vi "AutoWfmToSpreadsheet_2019.vi"() -> ()   [LabVIEW 2019]
uses:
  <vilib>/Waveform/WDTFileIO.llb/Read Waveform from File.vi
  <vilib>/Waveform/WDTOps.llb/WDT Index Channel DBL.vi
  <vilib>/Waveform/WDTFileIO.llb/Export Waveforms To Spreadsheet File (1D).vi
panel:
  out "?":string
  in  "Path":i32
  in  "Path":string[](array[string])
  out "?":string
  out "Sinal adquirido":waveform(dbl)(graph)
  in  "?":bool
  in  "Escolher arquivo":i32
  out "Sinal de Referência":waveform(dbl)(graph)
  in  "V para Exportar/ F para Visualizar":bool
  out "result string":string
  out "element":string
  out "Numeric":i32
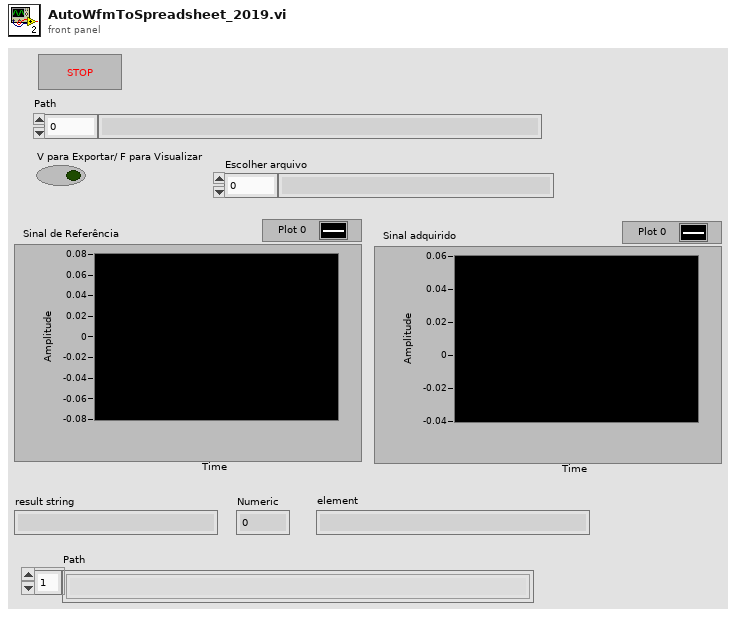
[diagram p1: front panel]
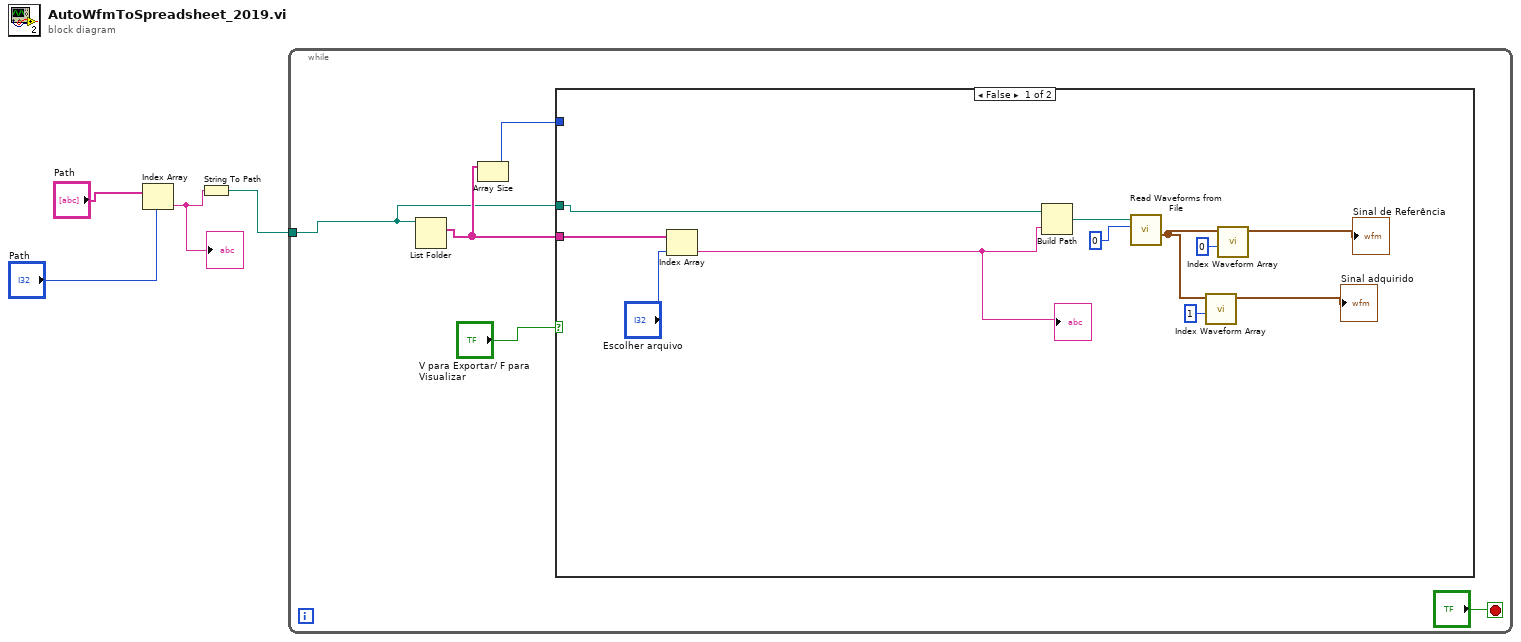
[diagram p0: block diagram]
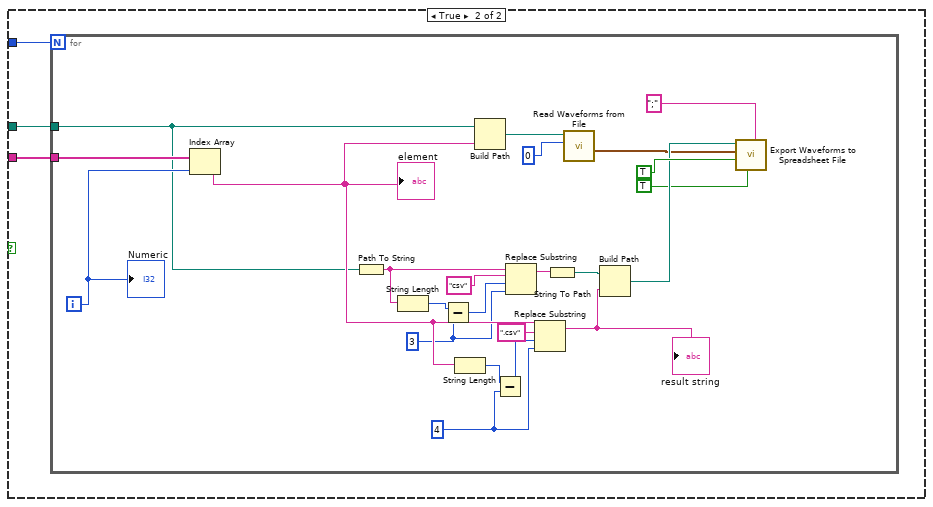
[diagram p2: hidden frame]
diagram:
  n1 = Index Array(array="Path", index="Path") -> (element=w1:string)
  "?" <- w1
  n2 = String To Path(string=w1) -> (path=w4:path)
  n3 = while {
    tunnel: w4 -> [w5]
    stop <- "?" stop-if-true
    n4 = List Folder(path=w5) -> (filenames=w9:string[])  [unwired: 3 in, 3 out]
    n5 = Array Size(array=w9) -> (size(s)=w8:i32)
    n6 = case shown="False" "V para Exportar/ F para Visualizar" {
      tunnel: w9 -> [w18 w23]
      tunnel: w8 -> [_ w22]
      tunnel: w5 -> [w10 w21]
      frame False {
        n7 = Index Array(array=w18, index="Escolher arquivo") -> (element=w13:string)
        "?" <- w13
        n8 = Build Path(base path=w10, name or relative path=w13) -> (appended path=w20:path)
        n9 = call-poly <vilib>:"Read Waveforms from File.vi"("offset (records:0)"=0, "file path (dialog if empty)"=w20) -> ("all waveforms in record"=w14:waveform(dbl)[])  [unwired: 4 in, 3 out]
        n10 = call-poly <vilib>:"Index Waveform Array.vi"("index"=1, "waveform array"=w14) -> ("waveform"=→"Sinal adquirido":waveform(dbl))  [unwired: 8 in, 1 out]
        n11 = call-poly <vilib>:"Index Waveform Array.vi"("index"=0, "waveform array"=w14) -> ("waveform"=→"Sinal de Referência":waveform(dbl))  [unwired: 8 in, 1 out]
      }
      frame True {
        n12 = for {
          N: w22 -> [_]
          tunnel: w23 -> [w46]
          tunnel: w21 -> [w31]
          i -> [w45]
          w26 = 3 ("y")
          w35 = 4 ("length (len. of substring)")
          n13 = Index Array(array=w46, index=w45) -> (element=w36:string)
          "element" <- w36
          n14 = Path To String(path=w31) -> (string=w29:string)
          n15 = String Length(string=w29) -> (length=w28:i32)
          n16 = Subtract(x=w28, y=w26) -> (x-y=w27:i32)
          n17 = String Length(string=w36) -> (length=w34:i32)
          n18 = Build Path(base path=w31, name or relative path=w36) -> (appended path=w43:path)
          n19 = Subtract(x=w34, y=w35) -> (x-y=w33:i32)
          n20 = Replace Substring(2:w26, 3:w27, 4:"csv" ("substring (\"\")"), 5:w29) -> (1:w25:string)  [unwired: 1 out]
          n21 = Replace Substring(2:w35, 3:w33, 4:".csv" ("substring (\"\")"), 5:w36) -> (1:w37:string)  [unwired: 1 out]
          "result string" <- w37
          n22 = String To Path(string=w25) -> (path=w24:path)
          n23 = call-poly <vilib>:"Read Waveforms from File.vi"("offset (records:0)"=0, "file path (dialog if empty)"=w43) -> ("all waveforms in record"=w32:waveform(dbl)[])  [unwired: 4 in, 3 out]
          n24 = Build Path(base path=w24, name or relative path=w37) -> (appended path=w40:path)
          n25 = call-poly <vilib>:"Export Waveforms to Spreadsheet File.vi"("delimiter (Tab)"=";", "append to file? (new file:F)"=TRUE, "multiple time columns? (single:F)"=TRUE, "waveforms"=w32, "file path (dialog if empty)"=w40) -> ()  [unwired: 5 in, 2 out]
          "Numeric" <- w45
        }
      }
    }
  }
